vi "Download Array.vi"(8 "error in":errorcluster, 10 "Data":u8[](array[numeric]) format="%.0x", 11 "Service Data Object in":refnum<class "Service Data Object.lvclass">) -> (0 "error out":errorcluster, 2 "CANopen Message out":refnum<class "CANopen Request Message.lvclass">, 3 "Service Data Object out":refnum<class "Service Data Object.lvclass">)   [LabVIEW 2024, in "CANopen Master.lvlib" / "Service Data Object.lvclass"]
uses:
  Service Data Object.lvclass
  Service Data Object.lvclass/Service Data Object.ctl
  CANopen/FunctionCode.ctl
  CANopen Master.lvlib
  CANopen Message/CANopen Message.lvclass
  CANopen Request/CANopen Request Message.lvclass
  D:/git/CANopen-XNET/CANopen Message/CANopen Message.lvclass
  D:/git/CANopen-XNET/CANopen Request/CANopen Request Message.lvclass
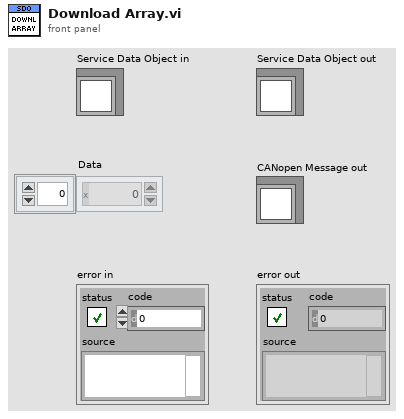
[diagram p1: front panel]
types:
  T1 = typedef "CANopen Master.lvlib/FunctionCode.ctl" = u16
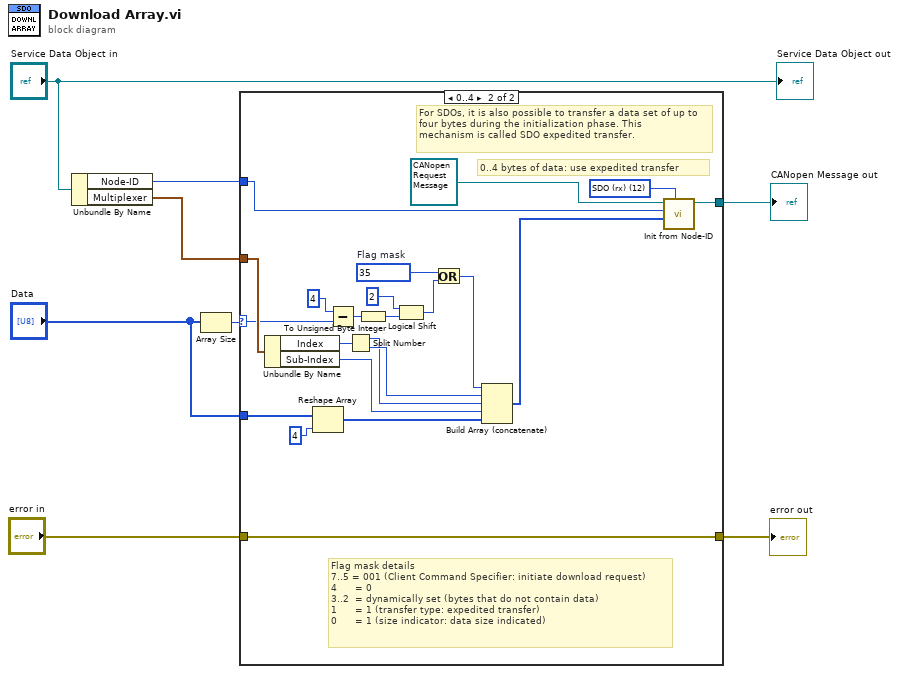
[diagram p0: block diagram]
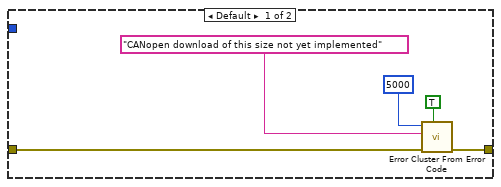
[diagram p2: hidden frame]
diagram:
  n1 = Unbundle By Name("Service Data Object in") -> ("Node-ID"=w2:u8, "Multiplexer"=w6:cluster{"Index":u16, "Sub-Index":u8})
  n2 = Array Size(array="Data") -> (size(s)=w8:i32)
  n3 = case shown="0..4" w8 {
    selector: w8 -> [_ w23]
    tunnel: [w13 w15] -> w3
    tunnel: "error in" -> [w10 w15]
    tunnel: "Data" -> [_ w27]
    tunnel: w6 -> [_ w35]
    tunnel: w2 -> [_ w19]
    tunnel: [_ w16] -> w1
    frame Default {
      n4 = call <vilib>:"Error Cluster From Error Code.vi"("show call chain? (False)"=TRUE, "error in (no error)"=w10, "error message (\"\")"="CANopen download of this size not yet implemented" ("source"), "error code (0)"=5000) -> ("error out"=w13:errorcluster)  [unwired: 5 in]
    }
    frame 0..4 {
      w17 = T1 12 items=["EMCY"=1, "PDO1 (tx)"=3, "PDO1 (rx)"=4, "PDO2 (tx)"=5, "PDO2 (rx)"=6, "PDO3 (tx)"=7, "PDO3 (rx)"=8, "PDO4 (tx)"=9, "PDO4 (rx)"=10, "SDO (tx)"=11, "SDO (rx)"=12, "NMT error control"=14] ("Function code")
      w28 = u8 35  # Flag mask
      # "For SDOs, it is also possible to transfer a data set of up to four bytes during the initialization phase. This \nmechanism is called SDO expedited transfer."
      # "Flag mask details\n7..5 = 001 (Client Command Specifier: initiate download request)\n4      = 0\n3..2  = dynamically set (bytes that do not contain data)\n1      = 1 (transfer type: expedited transfer)\n0      = 1 (size indicator: data size indicated)"
      # "0..4 bytes of data: use expedited transfer"
      n5 = Unbundle By Name(w35) -> ("Index"=w34:u16, "Sub-Index"=w31:u8)
      n6 = Reshape Array(w27, 4 ("y")) -> (w26:u8[])
      n7 = Subtract(x=4 ("y"), y=w23) -> (x-y=w24:i32)
      n8 = Split Number(x=w34) -> (hi(x)=w32:u8, lo(x)=w33:u8)
      n9 = To Unsigned Byte Integer(number=w24) -> (unsigned 8bit integer=w22:u8)
      n10 = Logical Shift(y=i8 2, x=w22) -> (x << y=w21:u8)
      n11 = Or(x=w28, y=w21) -> (x .or. y?=w29:u8)
      n12 = Build Array (concatenate)(w29, w33, w32, w31, w26) -> (w18:u8[])
      n13 = call "Init from Node-ID.vi"("Function code"=w17, "Data"=w18, "Node-ID"=w19, "CANopen Message in"=refnum<class "CANopen Request Message.lvclass"> refnum ("CANopen Master.lvlib:CANopen Request Message.lvclass")) -> ("CANopen Message in"=w16:refnum<class "CANopen Request Message.lvclass">)  [unwired: 7 in]
    }
  }
  "error out" <- w3
  "CANopen Message out" <- w1
  "Service Data Object out" <- "Service Data Object in"
